vi "IconPhraseMatch.vi"(10 "Array 3":i32[](array[numeric]), 11 "Array in":string[](array[string])) -> (3 "Array out":string[](array[string]))   [LabVIEW 2015]
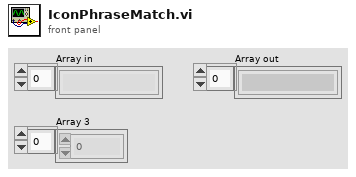
[diagram p1: front panel]
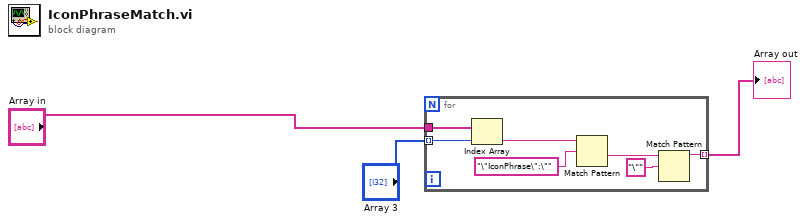
[diagram p0: block diagram]
diagram:
  n1 = for {
    tunnel: "Array 3" -> [w10] mode=indexing
    tunnel: [w5] -> w2 mode=indexing
    tunnel: "Array in" -> [w4]
    n2 = Index Array(array=w4, index=w10) -> (element=w9:string)
    n3 = Match Pattern(string=w9, regular expression="\"IconPhrase\":\"") -> (after substring=w7:string)  [unwired: 1 in, 3 out]
    n4 = Match Pattern(string=w7, regular expression="\"") -> (before substring=w5:string)  [unwired: 1 in, 3 out]
  }
  "Array out" <- w2
